vi "命令输出.vi"(8 "error in (no error)":errorcluster caption="错误输入（无错误）", 11 "Cleaningcycle 输入":refnum<class "Cleaning cycle.lvclass">) -> (0 "error out":errorcluster caption="错误输出", 2 "命令":cluster{"触发":bool, "周期项":T1}[](array[cluster]), 3 "Cleaningcycle 输出":refnum<class "Cleaning cycle.lvclass">)   [LabVIEW 2022 SP3, in "Cleaning cycle.lvclass"]
uses:
  Cleaning cycle.lvclass
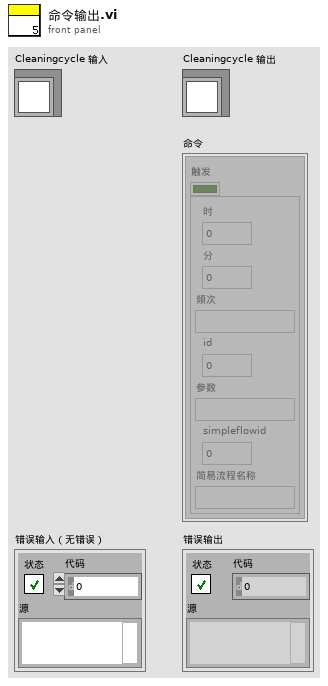
[diagram p1: front panel]
types:
  T1 = typedef "Cleaning cycle.lvclass/周期项.ctl" = cluster{"时":i32, "分":i32, "频次":string, "id":i32, "参数":string, "simpleflowid":i32, "简易流程名称":string}
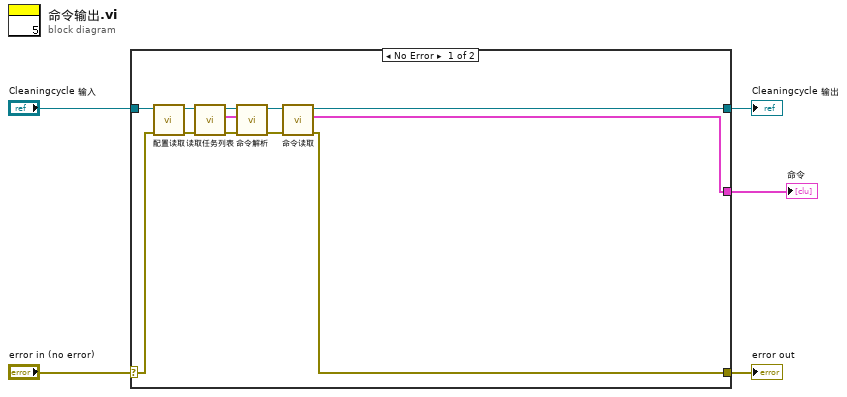
[diagram p0: block diagram]
diagram:
  n1 = case shown="No Error" "error in (no error)" {
    selector: "error in (no error)" -> [w7 w19]
    tunnel: [w11 w19] -> w4
    tunnel: [w12 w18] -> w2
    tunnel: "Cleaningcycle 输入" -> [w6 w18]
    tunnel: [w10 _] -> w1
    frame No Error {
      n2 = call "配置读取.vi"("error in (no error)"=w7, "Cleaningcycle 输入"=w6) -> ("error out"=w8:errorcluster, "Cleaningcycle 输出"=w9:refnum<class "Cleaning cycle.lvclass">)  [unwired: 8 in]
      n3 = call "读取任务列表.vi"("error in (no error)"=w8, "Cleaningcycle 输入"=w9) -> ("error out"=w15:errorcluster, "输出簇"=w16:cluster{"启用":bool, T1[]}, "Cleaningcycle 输出"=w17:refnum<class "Cleaning cycle.lvclass">)  [unwired: 7 in]
      n4 = call "命令解析.vi"("error in (no error)"=w15, "任务列表解析"=w16, "Cleaningcycle 输入"=w17) -> ("error out"=w13:errorcluster, "Cleaningcycle 输出"=w14:refnum<class "Cleaning cycle.lvclass">)  [unwired: 7 in]
      n5 = call-dynamic "命令读取.vi"("error in (no error)"=w13, "Cleaningcycle 输入"=w14) -> ("error out"=w11:errorcluster, "命令"=w10:cluster{"触发":bool, "周期项":T1}[], "Cleaningcycle 输出"=w12:refnum<class "Cleaning cycle.lvclass">)  [unwired: 7 in]
    }
    frame Error {
    }
  }
  "error out" <- w4
  "Cleaningcycle 输出" <- w2
  "命令" <- w1
